vi "Distance.vi"(8 "error in (no error)":errorcluster, 10 "Waveform in":waveform(dbl), 11 "RFID system in":refnum<class "RFID system.lvclass">) -> (0 "error out":errorcluster, 2 "Waveform out":waveform(dbl), 3 "RFID system out":refnum<class "RFID system.lvclass">)   [LabVIEW 2019, in "RFID system.lvclass"]
uses:
  RFID system.lvclass
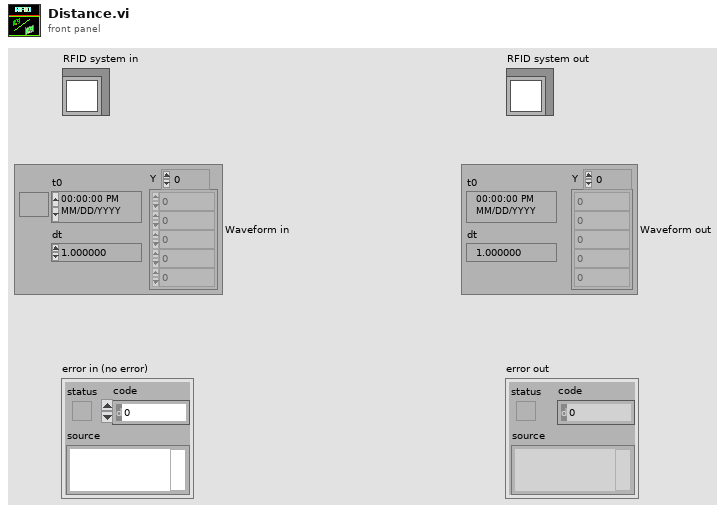
[diagram p1: front panel]
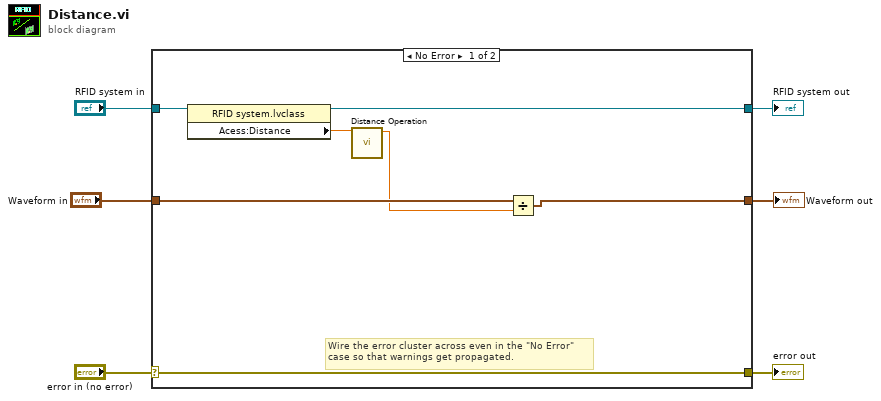
[diagram p0: block diagram]
diagram:
  n1 = case shown="No Error" "error in (no error)" {
    selector: "error in (no error)" -> [w12 w16]
    tunnel: [w12 w16] -> w5
    tunnel: [w11 w15] -> w3
    tunnel: "RFID system in" -> [w13 w15]
    tunnel: [w7 w14] -> w1
    tunnel: "Waveform in" -> [w9 w14]
    frame No Error {
      # "Wire the error cluster across even in the \"No Error\"\ncase so that warnings get propagated."
      n2 = property class="RFID system.lvclass"(reference=w13) -> (reference out=w11:refnum<class "RFID system.lvclass">, "Acess:Distance"=w10:dbl)  [unwired: 1 in, 1 out]
      n3 = call "Distance Operation.vi"("мм"=w10) -> ("ослабление"=w8:dbl)  [unwired: 10 in]
      n4 = Divide(x=w9, y=w8) -> (x/y=w7:waveform(dbl))
    }
    frame Error {
    }
  }
  "error out" <- w5
  "RFID system out" <- w3
  "Waveform out" <- w1
